vi "FlushShow.vi"(0 "引用输出":refnum<vi>) -> (14 "引用输出":refnum<vi>, 15 "所有连接名称":string[](array[string]))   [LabVIEW 2019]
uses:
  02 Mode/TCPServerMode/TCPServerClass.lvclass
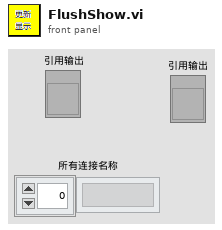
[diagram p1: front panel]
types:
  T1 = typedef "串口枚举.ctl" = enum16{"ini", "增", "删", "查", "改"}
  T2 = map{string, refnum<class "TCPClientClass.lvclass">}
  T3 = map{string, refnum<class "TCPServerClass.lvclass">}
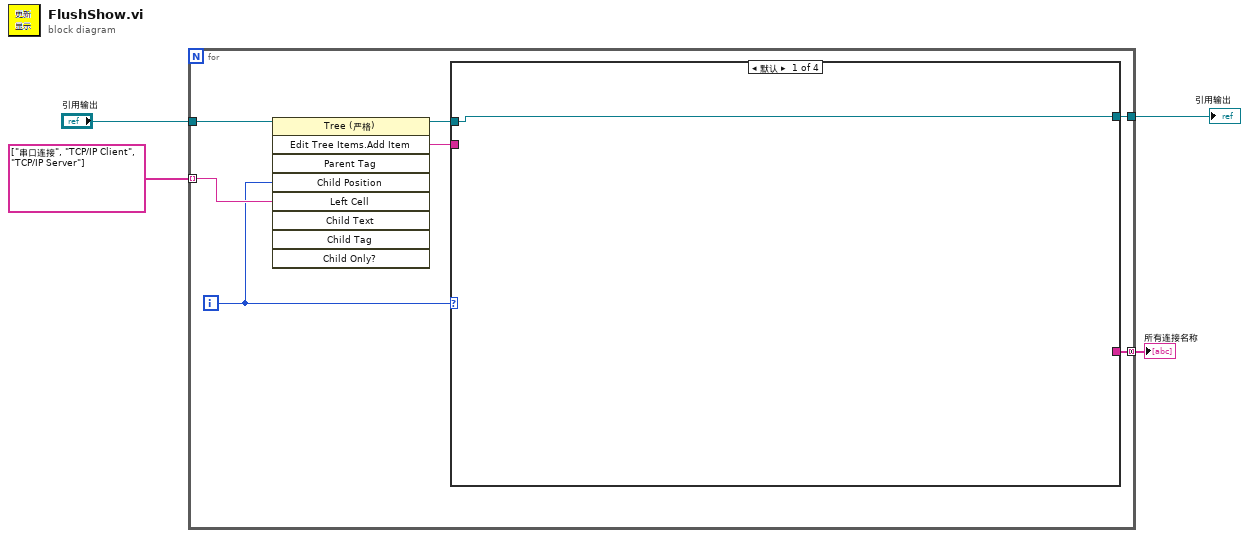
[diagram p0: block diagram]
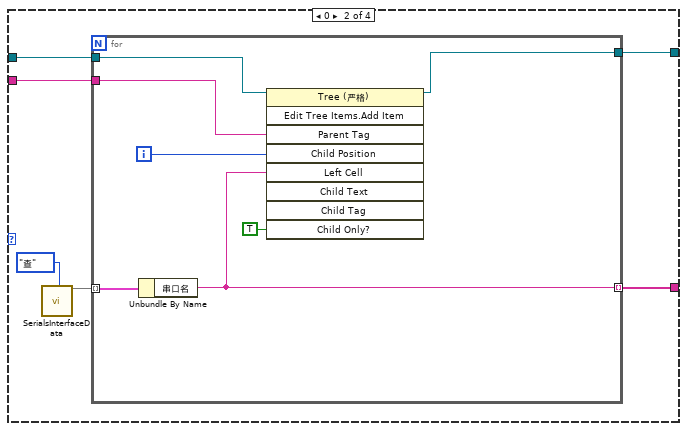
[diagram p2: hidden frame]
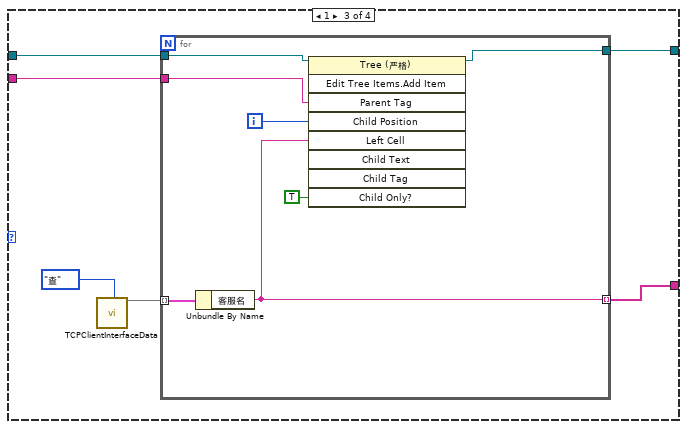
[diagram p3: hidden frame]
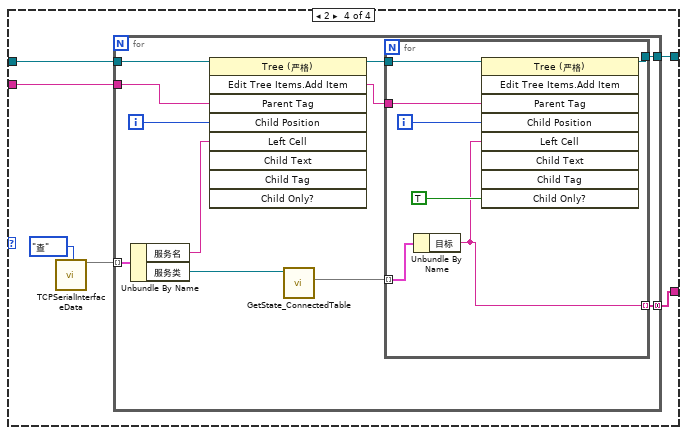
[diagram p4: hidden frame]
diagram:
  n1 = for {
    tunnel: string[] ["串口连接", "TCP/IP Client", "TCP/IP Server"] -> [w10] mode=indexing
    tunnel: "引用输出" -> [w11]
    tunnel: [w6] -> w2 mode=concatenating
    tunnel: [w5] -> w1
    i -> [w9]
    n2 = invoke class="Tree (严格)" method="Edit Tree Items.Add Item"(reference=w11, "Child Position"=w9, "Left Cell"=w10) -> (reference out=w7:refnum<vi>, "Edit Tree Items:Add Item"=w8:string)  [unwired: 6 in, 7 out]
    n3 = case shown="默认" w9 {
      tunnel: w8 -> [_ w18 w30 w43]
      tunnel: w7 -> [w12 w17 w31 w44]
      tunnel: [_ w14 w27 w40] -> w6
      tunnel: [w12 w13 w26 w39] -> w5
      frame Default {
      }
      frame 0 {
        n4 = call "SerialsInterfaceData.vi"("串口枚举"=串口枚举."查") -> ("串口表"=w15:map{string, refnum<class "SerialClass.lvclass">})  [unwired: 17 in, 1 out]
        n5 = for {
          tunnel: w15 -> [w25] mode=indexing
          tunnel: w18 -> [w23]
          tunnel: w17 -> [w21]
          tunnel: [w20] -> w14 mode=indexing
          tunnel: [w19] -> w13
          i -> [w24]
          n6 = Unbundle By Name(w25) -> ("串口名"=w20:string)
          n7 = invoke class="Tree (严格)" method="Edit Tree Items.Add Item"(reference=w21, "Parent Tag"=w23, "Child Position"=w24, "Left Cell"=w20, "Child Only?"=TRUE ("仅作为子项？")) -> (reference out=w19:refnum<vi>)  [unwired: 4 in, 8 out]
        }
      }
      frame 1 {
        n8 = call "TCPClientInterfaceData.vi"("客服接口枚举"=enum16{"ini", "增", "删", "查", "改"}."查") -> ("客服表"=w28:T2)  [unwired: 17 in, 1 out]
        n9 = for {
          tunnel: w31 -> [w38]
          tunnel: w30 -> [w37]
          tunnel: w28 -> [w36] mode=indexing
          tunnel: [w33] -> w27 mode=indexing
          tunnel: [w32] -> w26
          i -> [w35]
          n10 = Unbundle By Name(w36) -> ("客服名"=w33:string)
          n11 = invoke class="Tree (严格)" method="Edit Tree Items.Add Item"(reference=w38, "Parent Tag"=w37, "Child Position"=w35, "Left Cell"=w33, "Child Only?"=TRUE ("仅作为子项？")) -> (reference out=w32:refnum<vi>)  [unwired: 4 in, 8 out]
        }
      }
      frame 2 {
        n12 = call "TCPSerialInterfaceData.vi"("客服接口枚举"=enum16{"ini", "增", "删", "查", "改"}."查") -> ("服务表"=w41:T3)  [unwired: 17 in, 1 out]
        n13 = for {
          tunnel: w44 -> [w54]
          tunnel: w43 -> [w53]
          tunnel: w41 -> [w55] mode=indexing
          tunnel: [w46] -> w40 mode=concatenating
          tunnel: [w45] -> w39
          i -> [w52]
          n14 = Unbundle By Name(w55) -> ("服务名"=w51:string, "服务类"=w48:refnum<class "TCPServerClass.lvclass">)
          n15 = invoke class="Tree (严格)" method="Edit Tree Items.Add Item"(reference=w54, "Parent Tag"=w53, "Child Position"=w52, "Left Cell"=w51) -> (reference out=w50:refnum<vi>, "Edit Tree Items:Add Item"=w49:string)  [unwired: 5 in, 7 out]
          n16 = call-dynamic "GetState_ConnectedTable.vi"("TCPServerClass输入"=w48) -> ("连接端ID表"=w47:map{string, refnum<k5>})  [unwired: 8 in, 2 out]
          n17 = for {
            tunnel: w50 -> [w62]
            tunnel: w49 -> [w61]
            tunnel: w47 -> [w58] mode=indexing
            tunnel: [w57] -> w46 mode=indexing
            tunnel: [w56] -> w45
            i -> [w60]
            n18 = Unbundle By Name(w58) -> ("目标"=w57:string)
            n19 = invoke class="Tree (严格)" method="Edit Tree Items.Add Item"(reference=w62, "Parent Tag"=w61, "Child Position"=w60, "Left Cell"=w57, "Child Only?"=TRUE ("仅作为子项？")) -> (reference out=w56:refnum<vi>)  [unwired: 4 in, 8 out]
          }
        }
      }
    }
  }
  "所有连接名称" <- w2
  "引用输出" <- w1
